vi "Get DAQmx DO Task Ref from DO IOName.vi"(8 "error in (no error)":errorcluster, 10 "DO IOName":string, 11 "DAQ":refnum<class "DAQ.lvclass">) -> (0 "error out":errorcluster, 2 "DAQmx DO Task":refnum<k21>, 3 "DAQ":refnum<class "DAQ.lvclass">)   [LabVIEW 2017, in "DAQ.lvclass"]
doc: "Developed by Kevin Thompson\nkevin@thompsonengineering.net\n\nCopyright 2018-2020\nThompson Engineering, LLC"
uses:
  DAQ.lvclass
  DAQ.lvclass/DAQ.ctl
  DataTypes/TD DO Channel--cluster.ctl
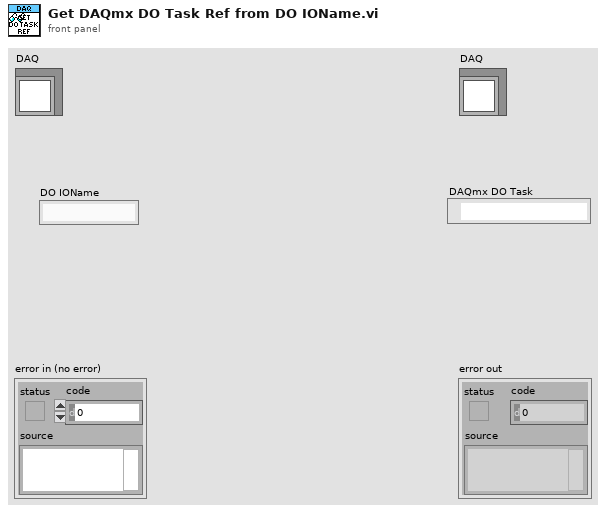
[diagram p1: front panel]
types:
  T1 = typedef "DAQ.lvclass/TD DO Channel--cluster.ctl" = cluster{"DevName":string, "IOName":string, "IOPath":string, "SchemName":string, "logic":enum16{"Lo", "Hi"}, "DAQmx Task":refnum<k21>}
  T2 = typedef "TD Dynamic CVT DVR--ref.ctl" = refnum<data-value>
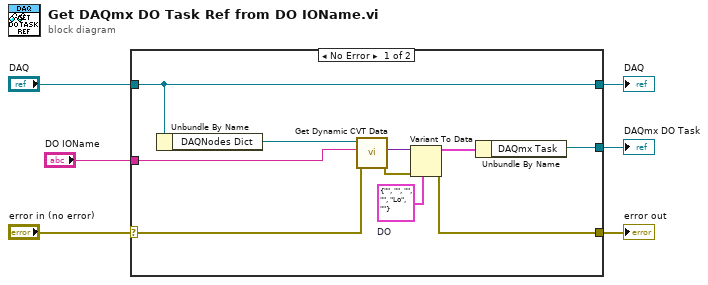
[diagram p0: block diagram]
diagram:
  n1 = case shown="No Error" "error in (no error)" {
    selector: "error in (no error)" -> [w14 w17]
    tunnel: [w13 w17] -> w5
    tunnel: [w16 w18] -> w3
    tunnel: "DAQ" -> [w16 w18]
    tunnel: "DO IOName" -> [w8 _]
    tunnel: [w9 _] -> w1
    frame No Error {
      w7 = T1 {"DevName"="", "IOName"="", "IOPath"="", "SchemName"="", "logic"=enum."Lo", "DAQmx Task"=""}  # DO
      n2 = Unbundle By Name(w16) -> ("DAQNodes Dict"=w15:T2)
      n3 = call <vilib>:"Get Dynamic CVT Data.vi"("error in (no error)"=w14, "DataName"=w8, "dCVT DVR"=w15) -> ("error out"=w12:errorcluster, "value"=w11:variant)  [unwired: 5 in, 2 out]
      n4 = Variant To Data(error in=w12, type=w7, Variant=w11) -> (data=w10:T1, error out=w13:errorcluster)
      n5 = Unbundle By Name(w10) -> ("DAQmx Task"=w9:refnum<k21>)
    }
    frame Error {
    }
  }
  "error out" <- w5
  "DAQ" <- w3
  "DAQmx DO Task" <- w1
